vi "Variant to Bool.vi"(10 "error in":errorcluster, 11 "data variant":variant) -> (2 "error out":errorcluster, 3 "data out":bool)   [LabVIEW 2018]
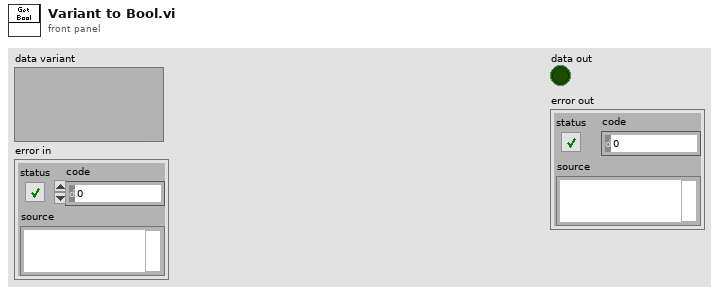
[diagram p1: front panel]
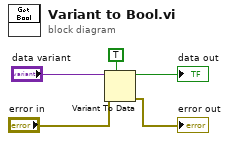
[diagram p0: block diagram]
diagram:
  n1 = Variant To Data(error in="error in", type=TRUE, Variant="data variant") -> (data=→"data out":bool, error out=→"error out":errorcluster)
